vi "Bone_Init.vi"(3 "error in":errorcluster, 4 "Task":enum16{"Init", "Close"}(ring), 5 "Connection in":T1) -> (0 "error out":errorcluster, 1 "String":string, 2 "Connection Out":T1)   [LabVIEW 2012]
uses:
  <userlib>/BotSpeak/VIs/SubVIs/CommState.ctl
  <userlib>/BotSpeak/VIs/Direct/BotSpeak_Control.ctl
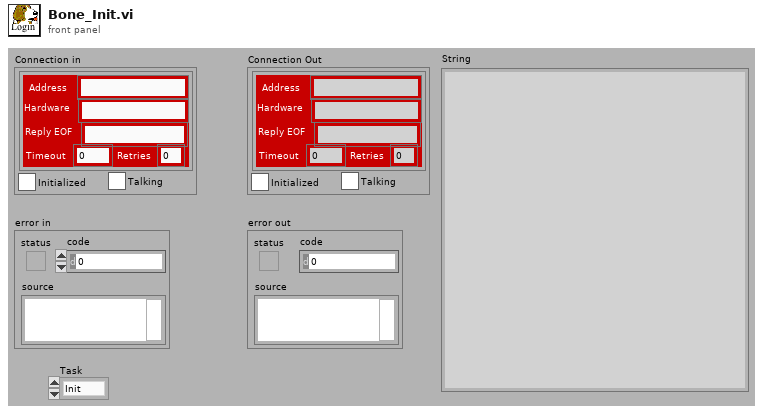
[diagram p1: front panel]
types:
  T1 = typedef "CommState.ctl" = cluster{"Bot Settings":T2, "Initialized":bool, "Talking":bool}
  T2 = typedef "BotSpeak_Control.ctl" = cluster{"Address":string, "Reply EOF":string, "Hardware":string, "Retries":i8, "Timeout":i32}
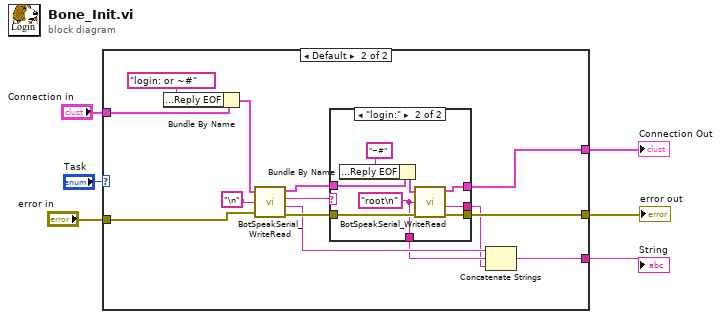
[diagram p0: block diagram]
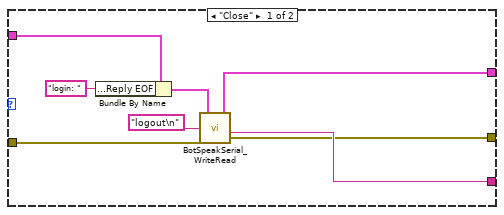
[diagram p2: hidden frame]
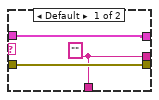
[diagram p3: hidden frame]
diagram:
  n1 = case shown="Default" "Task" {
    tunnel: [w12 w28] -> w6
    tunnel: [w10 w26] -> w5
    tunnel: "Connection in" -> [w9 w22]
    tunnel: [w13 w17] -> w3
    tunnel: "error in" -> [w11 w15]
    frame "Close" {
      n2 = Bundle By Name(cluster=w9, "Bot Settings.Reply EOF"="login: ") -> (w8:T1)
      n3 = call <userlib>:"BotSpeakSerial_WriteRead.vi"("error In"=w11, "To Write"="logout\n" ("String To Send"), "Connection In"=w8) -> ("error out"=w12:errorcluster, "Reply"=w13:string, "Connection Out"=w10:T1)  [unwired: 1 out]
    }
    frame Default {
      n4 = Bundle By Name(cluster=w22, "Bot Settings.Reply EOF"="login: or ~#" ("Status String")) -> (w23:T1)
      n5 = call <userlib>:"BotSpeakSerial_WriteRead.vi"("error In"=w15, "To Write"="\n" ("Status String"), "Connection In"=w23) -> ("error out"=w27:errorcluster, "Reply"=w20:string, "Reply EOF"=w16:string, "Connection Out"=w25:T1)
      n6 = case shown="\"login:\"" w16 {
        tunnel: [w30 w39] -> w28
        tunnel: w27 -> [w30 w38]
        tunnel: [w31 w37] -> w26
        tunnel: w25 -> [w31 w34]
        tunnel: [w29 w33] -> w19
        tunnel: [w29 w32] -> w18
        frame Default {
          w29 = "" ("Status String")
        }
        frame "login:" {
          w33 = "root\n" ("Status String")
          n7 = Bundle By Name(cluster=w34, "Bot Settings.Reply EOF"="~#" ("Status String")) -> (w36:T1)
          n8 = call <userlib>:"BotSpeakSerial_WriteRead.vi"("error In"=w38, "To Write"=w33, "Connection In"=w36) -> ("error out"=w39:errorcluster, "Reply"=w32:string, "Connection Out"=w37:T1)  [unwired: 1 out]
        }
      }
      n9 = Concatenate Strings(w20, w19, w18) -> (w17:string)
    }
  }
  "error out" <- w6
  "Connection Out" <- w5
  "String" <- w3
